vi "SelectAppRef.vi"(11 "Application in":refnum<vi>) -> (3 "Application out":refnum<vi>)   [LabVIEW 2013]
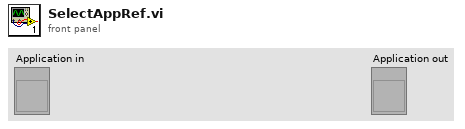
[diagram p1: front panel]
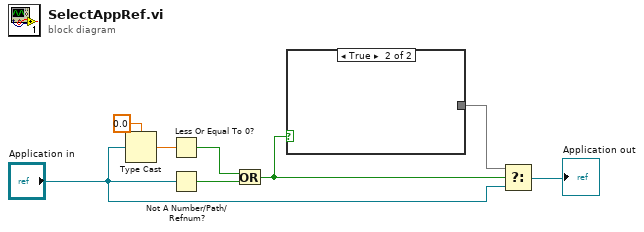
[diagram p0: block diagram]
diagram:
  n1 = Type Cast(type=0.0 ("x"), x="Application in") -> (*(type *) &x=w4:dbl)
  n2 = Less Or Equal To 0?(x=w4) -> (x <= 0?=w5:bool)
  n3 = Not A Number/Path/Refnum?(number/path/refnum="Application in") -> (NaN/Path/Refnum?=w7:bool)
  n4 = Or(x=w5, y=w7) -> (x .or. y?=w2:bool)
  n5 = case shown="True" w2 {
    tunnel: [_ _] -> w1
    frame False {
    }
    frame True {
    }
  }
  n6 = Select(t=w1, s=w2, f="Application in") -> (s? t:f=→"Application out":refnum<vi>)
